vi "VI Infomation RTM.vi"(8 "error in (no error)":errorcluster, 9 "Ctl Refnum":refnum<vi>, 10 "Menu Tag":string, 11 "Interface in":refnum<class "Interface.lvclass">) -> (0 "error out":errorcluster, 3 "Interface out":refnum<class "Interface.lvclass">)   [LabVIEW 2015, in "Interface.lvlib" / "Interface.lvclass"]
uses:
  Interface.lvclass
  Controls/VI Infomation.ctl
  Interface.lvlib
  Interface Messages/RTM Activated Msg/RTM Activated Msg.lvclass
  <vilib>/ActorFramework/Actor/Actor.lvclass
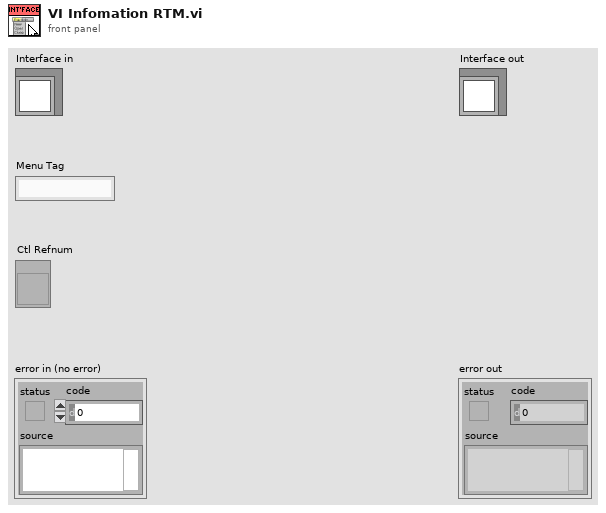
[diagram p1: front panel]
types:
  T1 = typedef "Interface.lvlib/VI Infomation.ctl" = cluster{"VI Name":string, "VI Description":string, "VI Icon":picture}
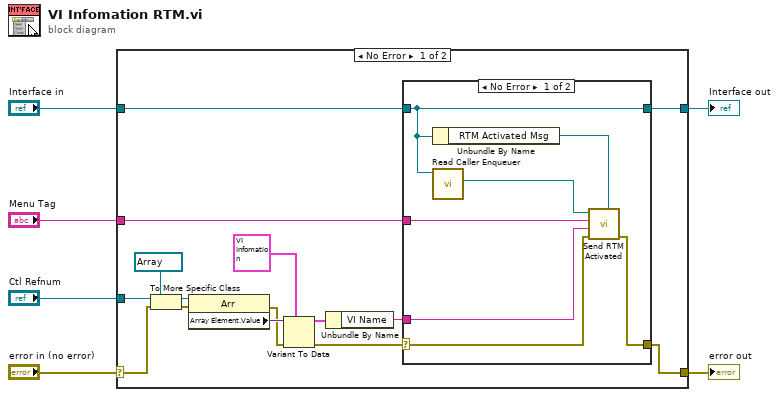
[diagram p0: block diagram]
diagram:
  n1 = case shown="No Error" "error in (no error)" {
    selector: "error in (no error)" -> [w14 w31]
    tunnel: [w7 w31] -> w5
    tunnel: [w10 w30] -> w3
    tunnel: "Interface in" -> [w9 w30]
    tunnel: "Menu Tag" -> [w8 _]
    tunnel: "Ctl Refnum" -> [w19 _]
    frame No Error {
      n2 = To More Specific Class(target class=refnum<vi> refnum ("Arr Refnum"), reference=w19, error in=w14) -> (specific class reference=w21:refnum<vi>, error out=w13:errorcluster)
      n3 = property class="Arr"(reference=w21, error in=w13) -> (error out=w12:errorcluster, "Array Element.Value"=w18:variant)  [unwired: 1 out]
      n4 = Variant To Data(error in=w12, type=T1 {"VI Name"="", "VI Description"="", "VI Icon"=bytes[0]} ("VI Infomation"), Variant=w18) -> (data=w16:T1, error out=w11:errorcluster)
      n5 = Unbundle By Name(w16) -> ("VI Name"=w15:string)
      n6 = case shown="No Error" w11 {
        selector: w11 -> [w23 _]
        tunnel: w15 -> [w26 _]
        tunnel: w8 -> [w27 _]
        tunnel: [w25 w29] -> w10
        tunnel: w9 -> [w25 w29]
        tunnel: [w22 _] -> w7
        frame No Error {
          n7 = Unbundle By Name(w25) -> ("RTM Activated Msg"=w28:refnum<class "RTM Activated Msg.lvclass">)
          n8 = call <vilib>:"Read Caller Enqueuer.vi"("Actor"=w25) -> ("Caller Enqueuer"=w24:refnum<class "Message Enqueuer.lvclass">)  [unwired: 10 in]
          n9 = call "Send RTM Activated.vi"("Message Type"=w28, "error in (no error)"=w23, "VI Name"=w26, "Tag"=w27, "Message Enqueuer"=w24) -> ("error out"=w22:errorcluster)  [unwired: 5 in, 1 out]
        }
        frame Error {
        }
      }
    }
    frame Error {
    }
  }
  "error out" <- w5
  "Interface out" <- w3
